vi "AI queue.vi"(5 "object":string="AZ1", 7 "date/time string":string, 8 "error in (no error)":errorcluster, 9 "analog parameters":dbl[](array[numeric]), 10 "AI table":string[](array[string]), 11 "AI_msg":refnum<queue>) -> (0 "error out":errorcluster)   [LabVIEW 2019, in "Inputs.lvlib"]
uses:
  Inputs.lvlib
  Database/PostgreSQL.lvlib
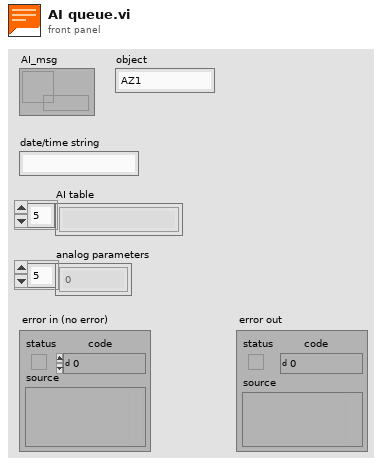
[diagram p1: front panel]
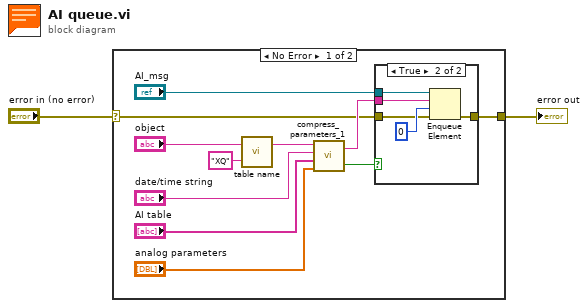
[diagram p0: block diagram]
diagram:
  n1 = case shown="No Error" "error in (no error)" {
    selector: "error in (no error)" -> [w3 w20]
    tunnel: [w9 w20] -> w2
    frame No Error {
      n2 = call "table name.vi"("postfix"="XQ", "object name"="object") -> ("table name"=w7:string)  [unwired: 1 in]
      n3 = call "compress_parameters_1.vi"("analog parameters"="analog parameters", "AI table"="AI table", "date/time string"="date/time string", "table"=w7) -> ("Data to write"=w4:bool, "parameters"=w13:string)
      n4 = case shown="True" w4 {
        tunnel: "AI_msg" -> [_ w18]
        tunnel: w13 -> [_ w17]
        tunnel: [w14 w16] -> w9
        tunnel: w3 -> [w14 w15]
        frame False {
        }
        frame True {
          n5 = Enqueue Element(queue=w18, element=w17, timeout in ms (-1)=0, error in (no error)=w15) -> (error out=w16:errorcluster)  [unwired: 2 out]
        }
      }
    }
    frame Error {
    }
  }
  "error out" <- w2
